vi "ACNET Devices Editor.vi"(8 "error in (no error)":errorcluster, 10 "ACNET Devices File":path) -> (0 "error out":errorcluster, 2 "ACNET Devices File (duplicate)":path)   [LabVIEW 2013]
uses:
  <vilib>/event_ctls.llb/eventvkey.ctl
  ACNET Monitor/ACNET Devices.lvclass
  ACNET Monitor/ACNET Device.lvclass
  ACNET Devices Editor.lvlib
  ACNET Monitor.lvlib
panel:
  in  "Load":bool
  in  "Save":bool
  in  "Remove":bool
  in  "New ACNET Device":T1
  in  "Add Device Limits":bool
  in  "stop":bool
  in  "ACNET Devices":i32[](listbox)
  # "ACNET Devices Editor.vi\nupdated on 5 Apr 2015\nby P. Lane"
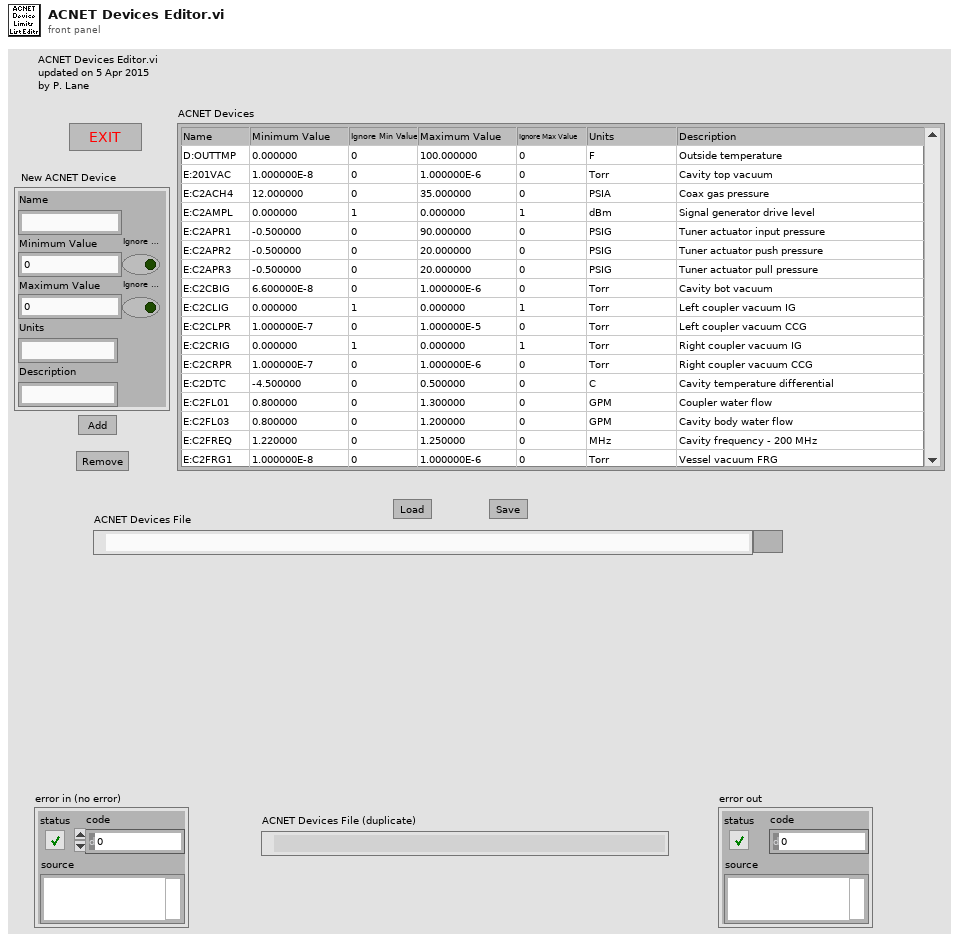
[diagram p1: front panel]
types:
  T1 = cluster{"Name":string, "Minimum Value":dbl, "Maximum Value":dbl, "Units":string, "Description":string, "Ignore Min Value":bool, "Ignore Max Value":bool}
  T2 = enum32{"Bad", "Idle", "Run top level", "Running"}
  T3 = typedef "eventvkey.ctl" = enum16{"ASCII", "Enter", "Return", "Shift", "Ctrl", "Alt", "Cmd", "Opt", "Caps", "NumLock", "Clear", "Break", "Up", "Down", "Left", "Right", "Insert", "Delete", "Home", "End", "PageUp", "PageDown", "Escape", "Help", "Pause", "ScrollLock", "F1", "F2", "F3", "F4", "F5", "F6", "F7", "F8", "F9", "F10", "F11", "F12", "F13", "F14", "F15", "F16", "F17", "F18", "F19", "F20", "F21", "F22", "F23", "F24", "Play", "VolumeUp", "VolumeDown", "Mute", "Two Byte Char"}
  T4 = cluster{"name":string, "minValue":dbl, "maxValue":dbl, "units":string, "description":string, "ignoreMinValue":bool, "ignoreMaxValue":bool}
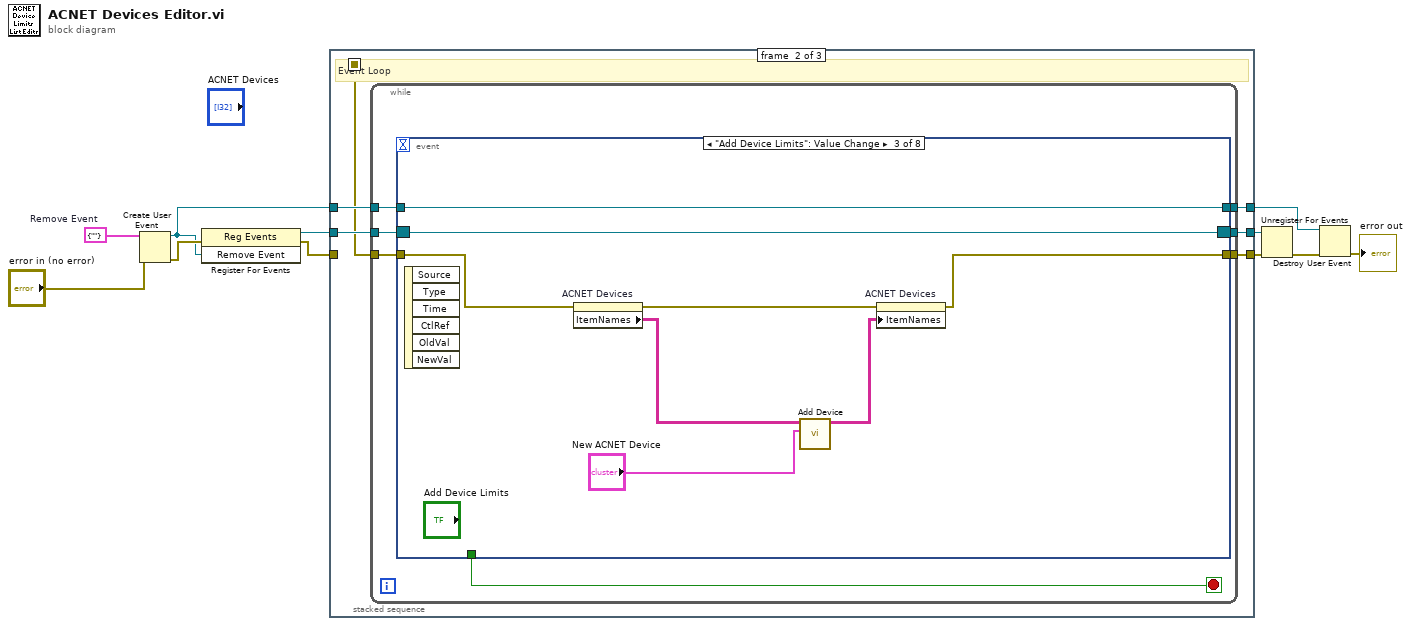
[diagram p0: block diagram]
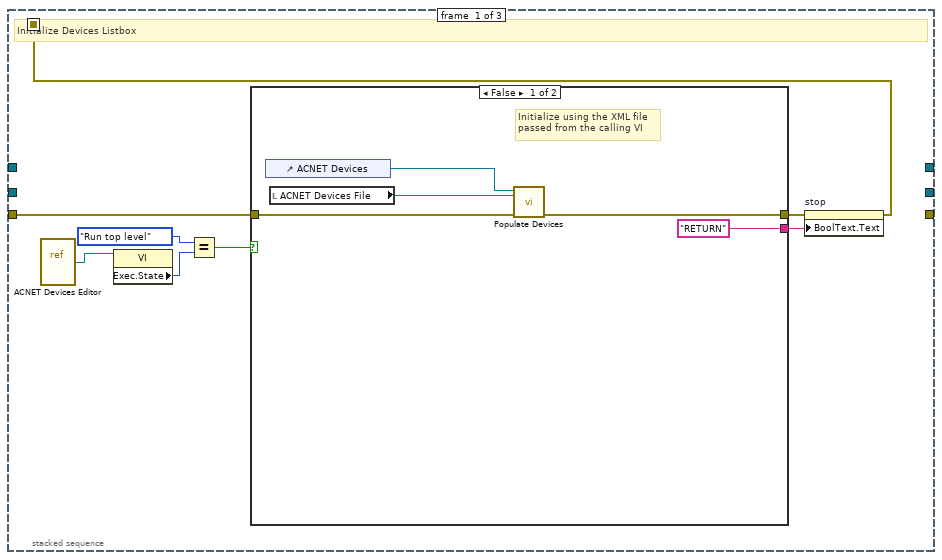
[diagram p2: hidden frame]
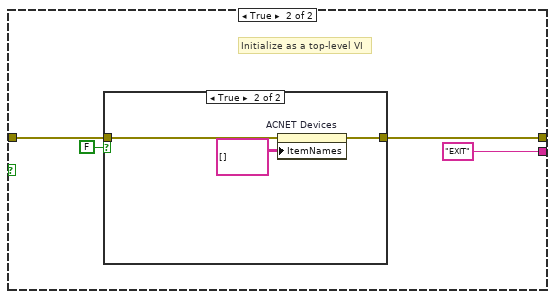
[diagram p3: hidden frame]
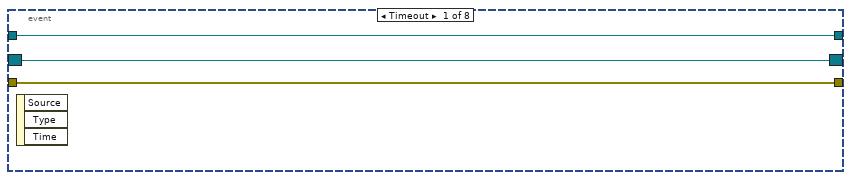
[diagram p5: hidden frame]
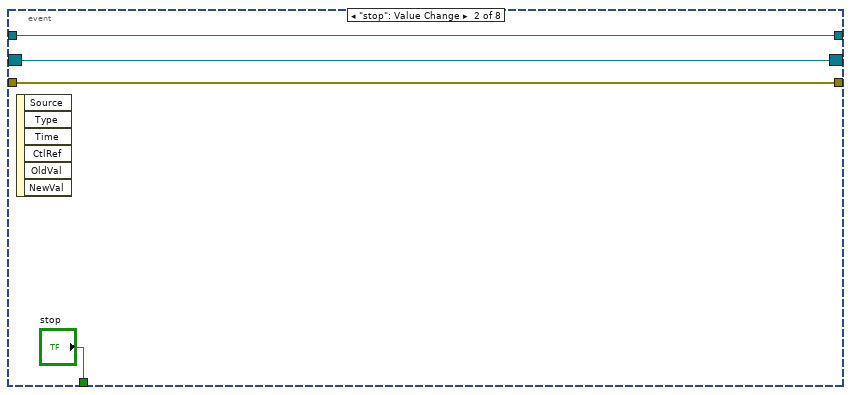
[diagram p6: hidden frame]
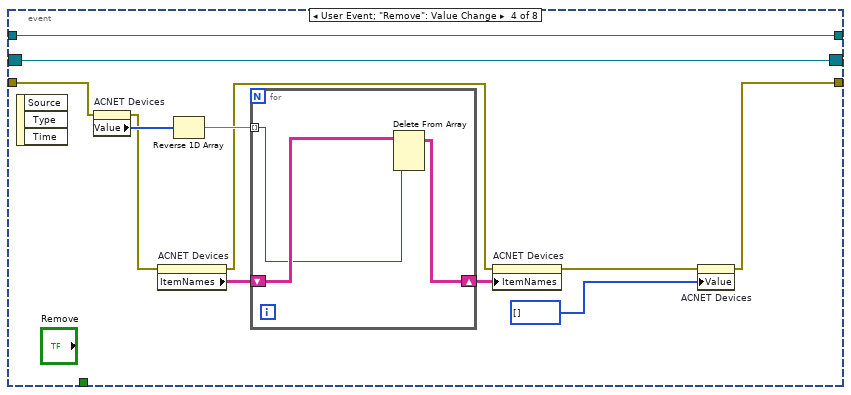
[diagram p7: hidden frame]
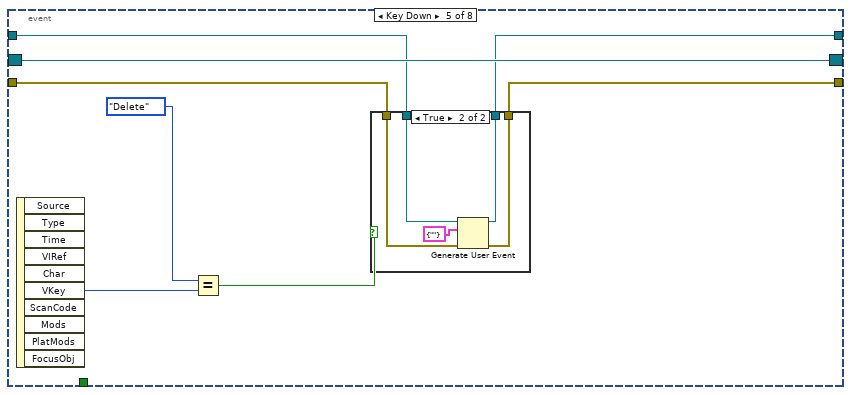
[diagram p8: hidden frame]
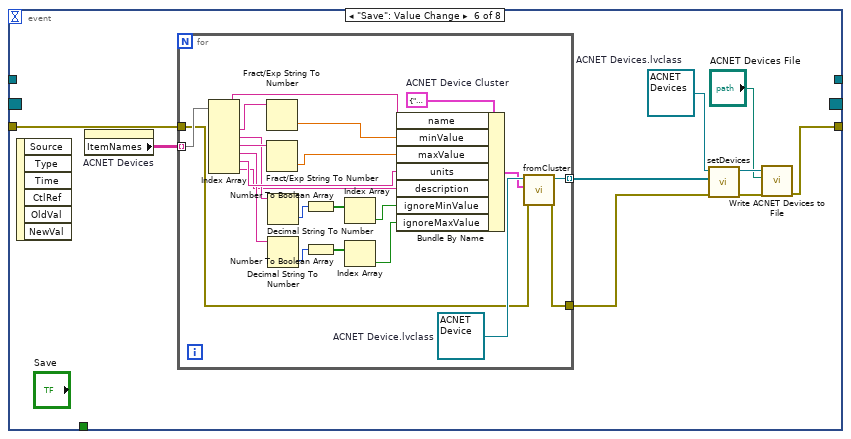
[diagram p10: hidden frame]
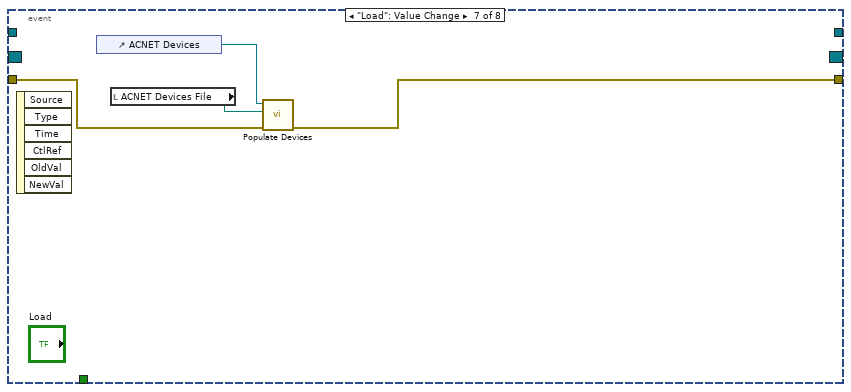
[diagram p11: hidden frame]
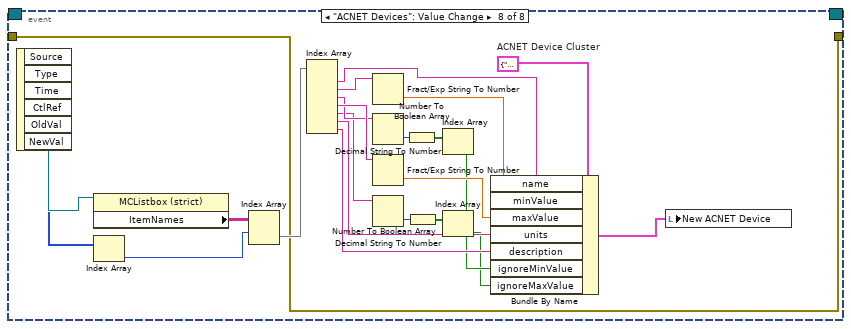
[diagram p12: hidden frame]
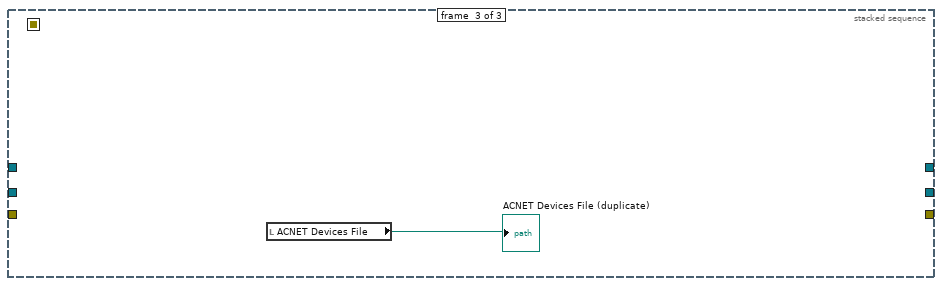
[diagram p13: hidden frame]
diagram:
  w10 = cluster{"string":string} {"string"=""}  # Remove Event
  n1 = Create User Event(user event datatype=w10, error in="error in (no error)") -> (user event=w3:refnum<user-event>, error out=w4:errorcluster)
  n2 = register-events(error in=w4, w3) -> (reference out=w11:refnum<event-registration>, error out=w8:errorcluster)  [unwired: 1 in]
  n3 = stacked-sequence {
    seq-local: [w12 _ _] -> [_ w33 _]
    tunnel: w11 -> [_ w38 _]
    tunnel: [_ w37 _] -> w9
    tunnel: w8 -> [w19 _ _]
    tunnel: [_ w36 _] -> w7
    tunnel: [_ w35 _] -> w5
    tunnel: w3 -> [_ w34 _]
    frame #0 {
      # "Initialize Devices Listbox"
      n4 = vi-ref "ACNET Devices Editor.vi"() -> (w16:refnum<vi>)
      n5 = property class="VI"(reference=w16) -> ("Exec.State"=w17:T2)  [unwired: 1 in, 2 out]
      n6 = Equal?(x=T2."Run top level" ("Execution:State"), y=w17) -> (x = y?=w15:bool)
      n7 = case shown="False" w15 {
        tunnel: w19 -> [w23 w28]
        tunnel: ["RETURN" "EXIT"] -> w14
        tunnel: [w20 w26] -> w13
        frame False {
          # "Initialize using the XML file\npassed from the calling VI"
          n8 = control-ref of="ACNET Devices"() -> (w24:refnum<vi>)
          n9 = local read "ACNET Devices File"() -> (w22:path)
          n10 = call "Populate Devices.vi"("error in (no error)"=w23, "List XML File"=w22, "MCListbox Refnum"=w24) -> ("error out"=w20:errorcluster)  [unwired: 8 in]
        }
        frame True {
          # "Initialize as a top-level VI"
          n11 = case shown="True" FALSE {
            tunnel: w28 -> [w29 w31]
            tunnel: [w29 w30] -> w26
            frame False {
            }
            frame True {
              n12 = property on="ACNET Devices" class="MCListbox (strict)"(error in=w31, "ItemNames"=string[][] [] ("Item Names")) -> (error out=w30:errorcluster)  [unwired: 1 in, 1 out]
            }
          }
        }
      }
      n13 = property on="stop" class="Bool"(error in=w13, "BoolText.Text"=w14) -> (error out=w12:errorcluster)  [unwired: 1 in, 1 out]
    }
    frame #1 {
      # "Event Loop"
      n14 = while {
        tunnel: w38 -> [w44]
        tunnel: [w43] -> w37
        tunnel: w33 -> [w42]
        tunnel: [w41] -> w36
        tunnel: w34 -> [w40]
        tunnel: [w39] -> w35
        stop <- w45 stop-if-true
        n15 = event shown="[2] \"Add Device Limits\": Value Change" {
          selector: w44 -> [w47 w50 w55 w62 w82 _ _ _]
          dyn-events: [w47 w50 w55 w62 w82 _ _ _] -> w43
          timeout: _ -> [_ _ _ _ _ _ _ _]
          tunnel: [_ "stop" _ _ _ _ _ _] -> w45
          tunnel: w42 -> [w48 w51 w58 w66 w79 w98 w124 w139]
          tunnel: [w48 w51 w56 w63 w78 w91 w123 w139] -> w41
          tunnel: w40 -> [w46 w49 w54 w61 w80 _ _ _]
          tunnel: [w46 w49 w54 w61 w77 _ _ _] -> w39
          event Timeout {
            n16 = event-data() -> ()  [unwired: 1 in, 3 out]
          }
          event "stop": Value Change {
            n17 = event-data() -> ()  [unwired: 1 in, 6 out]
          }
          event "Add Device Limits": Value Change {
            n18 = event-data() -> ()  [unwired: 1 in, 6 out]
            n19 = property on="ACNET Devices" class="MCListbox (strict)"(error in=w58) -> (error out=w57:errorcluster, "ItemNames"=w60:string[][])  [unwired: 1 in, 1 out]
            n20 = call "Add Device.vi"("New Device"="New ACNET Device", "ItemNames"=w60) -> ("Updated ItemNames"=w59:string[][])  [unwired: 9 in]
            n21 = property on="ACNET Devices" class="MCListbox (strict)"(error in=w57, "ItemNames"=w59) -> (error out=w56:errorcluster)  [unwired: 1 in, 1 out]
          }
          event User Event; "Remove": Value Change {
            n22 = event-data() -> ()  [unwired: 1 in, 3 out]
            n23 = property on="ACNET Devices" class="MCListbox (strict)"(error in=w66) -> (error out=w65:errorcluster, "Value"=w70:i32[])  [unwired: 1 in, 1 out]
            n24 = property on="ACNET Devices" class="MCListbox (strict)"(error in=w65) -> (error out=w64:errorcluster, "ItemNames"=w69:string[][])  [unwired: 1 in, 1 out]
            n25 = Reverse 1D Array(array=w70) -> (reversed array=w67:i32[])
            n26 = for {
              tunnel: w67 -> [w74] mode=indexing
              shift-right: [w73] -> w68
              shift-left: w69 -> [w75]
              n27 = Delete From Array(array=w75, index (row)=w74) -> (array with subset deleted=w73:string[][])  [unwired: 2 in, 1 out]
            }
            n28 = property on="ACNET Devices" class="MCListbox (strict)"(error in=w64, "ItemNames"=w68) -> (error out=w72:errorcluster)  [unwired: 1 in, 1 out]
            n29 = property on="ACNET Devices" class="MCListbox (strict)"(error in=w72, "Value"=i32[] [] ("Monitor List")) -> (error out=w63:errorcluster)  [unwired: 1 in, 1 out]
          }
          event Key Down {
            n30 = event-data() -> ("VKey"=w76:T3)  [unwired: 1 in, 9 out]
            n31 = Equal?(x=eventvkey."Delete" ("VKey"), y=w76) -> (x = y?=w81:bool)
            n32 = case shown="True" w81 {
              tunnel: w80 -> [w85 w90]
              tunnel: w79 -> [w84 w89]
              tunnel: [w84 w88] -> w78
              tunnel: [w85 w87] -> w77
              frame False {
              }
              frame True {
                n33 = Generate User Event(user event=w90, event data cluster=cluster{"string":string} {"string"=""} ("event data"), error in=w89) -> (user event out=w87:refnum<user-event>, error out=w88:errorcluster)  [unwired: 1 in]
              }
            }
          }
          event "Save": Value Change {
            w97 = refnum<class "ACNET Devices.lvclass"> refnum  # ACNET Devices.lvclass
            n34 = event-data() -> ()  [unwired: 1 in, 6 out]
            n35 = property on="ACNET Devices" class="MCListbox (strict)"() -> ("ItemNames"=w99:string[][])  [unwired: 2 in, 2 out]
            n36 = for {
              tunnel: w99 -> [w121] mode=indexing
              tunnel: [w115] -> w96 mode=indexing
              tunnel: w98 -> [w113]
              tunnel: [w114] -> w95
              w112 = T4 {"name"="", "minValue"=0.0, "maxValue"=0.0, "units"="", "description"="", "ignoreMinValue"=FALSE, "ignoreMaxValue"=FALSE}  # ACNET Device Cluster
              w116 = refnum<class "ACNET Device.lvclass"> refnum  # ACNET Device.lvclass
              n37 = Index Array(array=w121) -> (element #1=w119:string, element #2=w120:string, element #3=w108:string, element #4=w110:string, element #5=w101:string, element #6=w109:string, element #7=w100:string)  [unwired: 7 in]
              n38 = Fract/Exp String To Number(string=w120) -> (number=w118:dbl)  [unwired: 3 in, 1 out]
              n39 = Fract/Exp String To Number(string=w110) -> (number=w117:dbl)  [unwired: 3 in, 1 out]
              n40 = Decimal String To Number(string=w108) -> (number=w107:i32)  [unwired: 2 in, 1 out]
              n41 = Decimal String To Number(string=w101) -> (number=w104:i32)  [unwired: 2 in, 1 out]
              n42 = Number To Boolean Array(number=w107) -> (Boolean array=w106:bool[])
              n43 = Number To Boolean Array(number=w104) -> (Boolean array=w102:bool[])
              n44 = Index Array(array=w106) -> (element=w105:bool)  [unwired: 1 in]
              n45 = Index Array(array=w102) -> (element=w103:bool)  [unwired: 1 in]
              n46 = Bundle By Name(cluster=w112, "name"=w119, "minValue"=w118, "maxValue"=w117, "units"=w109, "description"=w100, "ignoreMinValue"=w105, "ignoreMaxValue"=w103) -> (w111:T4)
              n47 = call-dynamic "fromCluster.vi"("error in (no error)"=w113, "ACNET Device Cluster"=w111, "ACNET Device in"=w116) -> ("error out"=w114:errorcluster, "ACNET Device out"=w115:refnum<class "ACNET Device.lvclass">)  [unwired: 7 in]
            }
            n48 = call-dynamic "setDevices.vi"("error in (no error)"=w95, "Devices"=w96, "ACNET Devices in"=w97) -> ("error out"=w94:errorcluster, "ACNET Devices out"=w93:refnum<class "ACNET Devices.lvclass">)  [unwired: 7 in]
            n49 = call "Write ACNET Devices to File.vi"("error in (no error)"=w94, "XML File Path"="ACNET Devices File", "ACNET Devices in"=w93) -> ("error out"=w91:errorcluster)  [unwired: 7 in, 1 out]
          }
          event "Load": Value Change {
            n50 = event-data() -> ()  [unwired: 1 in, 6 out]
            n51 = control-ref of="ACNET Devices"() -> (w122:refnum<vi>)
            n52 = local read "ACNET Devices File"() -> (w125:path)
            n53 = call "Populate Devices.vi"("error in (no error)"=w124, "List XML File"=w125, "MCListbox Refnum"=w122) -> ("error out"=w123:errorcluster)  [unwired: 8 in]
          }
          event "ACNET Devices": Value Change {
            w137 = T4 {"name"="", "minValue"=0.0, "maxValue"=0.0, "units"="", "description"="", "ignoreMinValue"=FALSE, "ignoreMaxValue"=FALSE}  # ACNET Device Cluster
            n54 = event-data() -> ("CtlRef"=w148:refnum<vi>, "NewVal"=w147:i32[])  [unwired: 1 in, 4 out]
            n55 = property class="MCListbox (strict)"(reference=w148) -> ("ItemNames"=w146:string[][])  [unwired: 1 in, 2 out]
            n56 = Index Array(array=w147) -> (element=w145:i32)  [unwired: 1 in]
            n57 = Index Array(array=w146, index (row)=w145) -> (element=w140:string[])  [unwired: 1 in]
            n58 = Index Array(array=w140) -> (element #1=w143:string, element #2=w144:string, element #3=w133:string, element #4=w134:string, element #5=w132:string, element #6=w135:string, element #7=w136:string)  [unwired: 7 in]
            n59 = Fract/Exp String To Number(string=w144) -> (number=w142:dbl)  [unwired: 3 in, 1 out]
            n60 = Decimal String To Number(string=w133) -> (number=w131:i32)  [unwired: 2 in, 1 out]
            n61 = Fract/Exp String To Number(string=w134) -> (number=w141:dbl)  [unwired: 3 in, 1 out]
            n62 = Decimal String To Number(string=w132) -> (number=w130:i32)  [unwired: 2 in, 1 out]
            n63 = Number To Boolean Array(number=w131) -> (Boolean array=w129:bool[])
            n64 = Number To Boolean Array(number=w130) -> (Boolean array=w127:bool[])
            n65 = Index Array(array=w129) -> (element=w128:bool)  [unwired: 1 in]
            n66 = Index Array(array=w127) -> (element=w126:bool)  [unwired: 1 in]
            n67 = Bundle By Name(cluster=w137, "name"=w143, "minValue"=w142, "maxValue"=w141, "units"=w135, "description"=w136, "ignoreMinValue"=w128, "ignoreMaxValue"=w126) -> (w138:T4)
            n68 = local write "New ACNET Device"(w138) -> ()
          }
        }
      }
    }
    frame #2 {
      n69 = local read "ACNET Devices File"() -> (→"ACNET Devices File (duplicate)":path)
    }
  }
  n70 = Unregister For Events(event registration refnum=w9, error in=w7) -> (error out=w6:errorcluster)
  n71 = Destroy User Event(user event=w5, error in=w6) -> (error out=→"error out":errorcluster)
